vi "Read Done Flag.vi"(8 "error in (no error)":errorcluster, 11 "BasicTerminalBinding in":refnum<class "BasicTerminalBinding.lvclass">) -> (0 "error out":errorcluster, 2 "Done?":bool)   [LabVIEW 2017, in "TestViewables.lvlib" / "BasicTerminalBinding.lvclass"]
uses:
  BasicTerminalBinding.lvclass
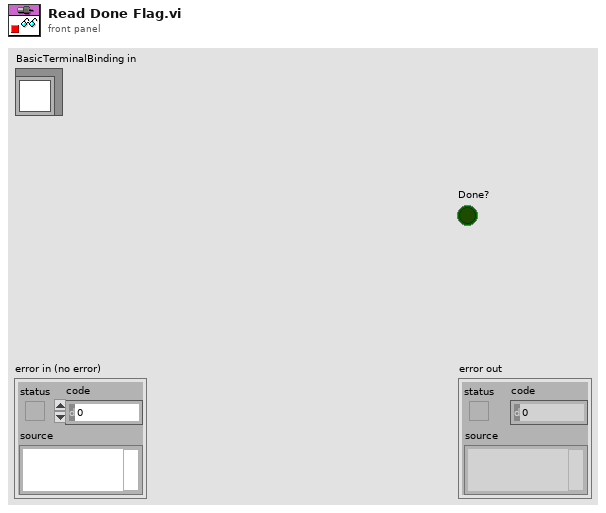
[diagram p1: front panel]
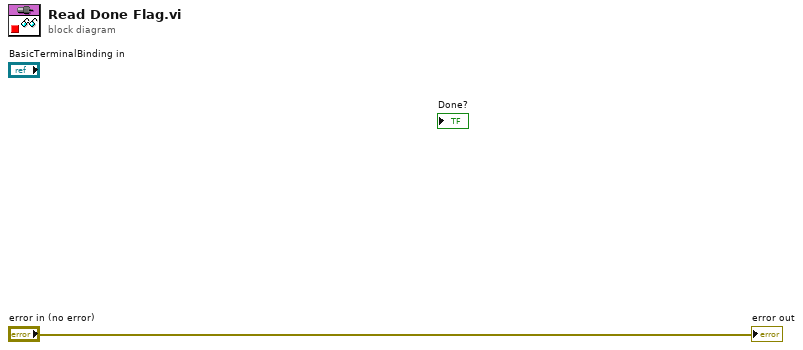
[diagram p0: block diagram]
diagram:
  "error out" <- "error in (no error)"
